vi "Database_User_Query.vi"(3 "error in (no error)":errorcluster, 4 "Column":string, 5 "Table":string, 6 "connection reference":T1) -> (0 "error out":errorcluster, 1 "size(s)":i32, 2 "connection reference 2":T1)   [LabVIEW 2015]
uses:
  <vilib>/addons/database/Connection.llb/Conn ObjectReference.ctl
  <vilib>/addons/database/Connection.llb/Conn Execute.vi
  <vilib>/addons/database/Recordset.llb/Rec Fetch Recordset Data (R).vi
  <vilib>/addons/database/Recordset.llb/Rec Destroy - Connection.vi
  <vilib>/addons/database/NI_Database_API.lvlib
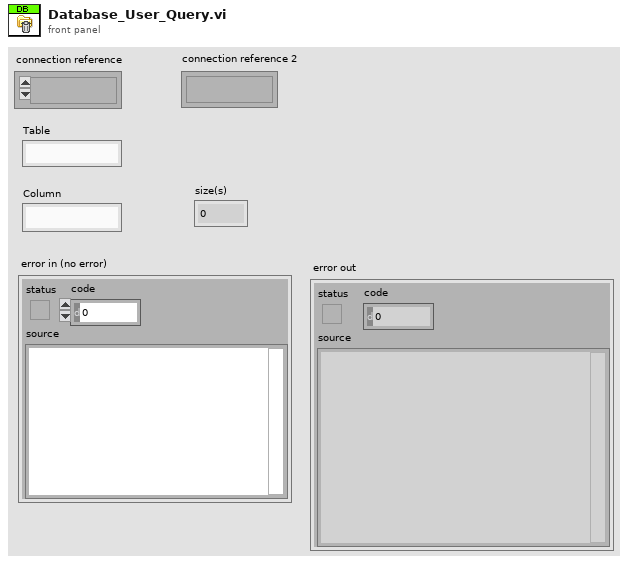
[diagram p1: front panel]
types:
  T1 = typedef "NI_Database_API.lvlib/Conn ObjectReference.ctl" = refnum<k1>
  T2 = typedef "NI_Database_API.lvlib/Rec ObjectReference.ctl" = refnum<k1>
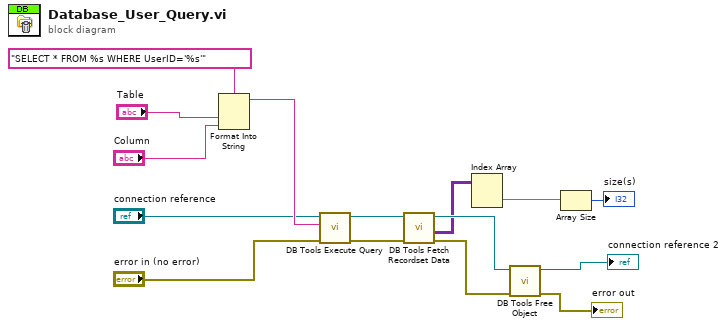
[diagram p0: block diagram]
diagram:
  n1 = Format Into String(format string="SELECT * FROM %s WHERE UserID='%s'" ("SQL query"), "Table", "Column") -> (resulting string=w13:string)  [unwired: 2 in, 1 out]
  n2 = call-poly <vilib>:"DB Tools Execute Query.vi"("error in (no error)"="error in (no error)", "SQL query"=w13, "connection reference"="connection reference") -> ("error out"=w11:errorcluster, "recordset reference"=w12:T2)  [unwired: 5 in]
  n3 = call-poly <vilib>:"DB Tools Fetch Recordset Data.vi"("error in (no error)"=w11, "recordset reference"=w12) -> ("error out"=w10:errorcluster, "recordset data"=w7:variant[][], "recordset reference out"=w8:T2)  [unwired: 3 in]
  n4 = Index Array(array=w7) -> (element=w6:variant[])  [unwired: 2 in]
  n5 = call-poly <vilib>:"DB Tools Free Object.vi"("error in (no error)"=w10, "recordset reference"=w8) -> ("error out"=→"error out":errorcluster, "connection reference"=→"connection reference 2":T1)  [unwired: 8 in]
  n6 = Array Size(array=w6) -> (size(s)=→"size(s)":i32)
